vi "Write Key Value Boolean.vi"(7 "Section Name":string, 8 "error in (no error)":errorcluster, 9 "Value":bool, 10 "Key Name":string, 11 "Ini-File in":refnum<class "Ini-File.lvclass">) -> (0 "error out":errorcluster, 2 "found":bool, 3 "Ini-File out":refnum<class "Ini-File.lvclass">)   [LabVIEW 2016, in "Configuration.lvlib" / "Ini-File.lvclass"]
doc: "Write boolean value."
uses:
  Ini-File.lvclass
  Ini-File.lvclass/Ini-File.ctl
  <vilib>/Utility/config.llb/Write Key (Boolean).vi
  <vilib>/Utility/config.llb/NI_LVConfig.lvlib
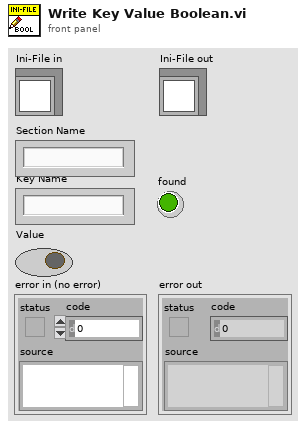
[diagram p1: front panel]
types:
  T1 = typedef "NI_LVConfig.lvlib/Config Data RefNum.ctl" = refnum<k1>
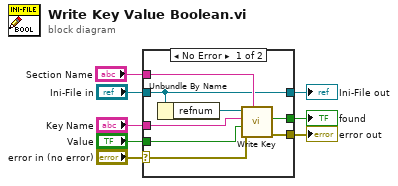
[diagram p0: block diagram]
diagram:
  n1 = case shown="No Error" "error in (no error)" {
    selector: "error in (no error)" -> [w9 w17]
    tunnel: "Ini-File in" -> [w10 w18]
    tunnel: "Section Name" -> [w15 _]
    tunnel: "Key Name" -> [w14 _]
    tunnel: "Value" -> [w13 _]
    tunnel: [w12 w17] -> w4
    tunnel: [w11 _] -> w3
    tunnel: [w10 w18] -> w2
    frame No Error {
      n2 = Unbundle By Name(w10) -> ("refnum"=w16:T1)
      n3 = call-poly <vilib>:"Write Key.vi"("section"=w15, "error in (no error)"=w9, "value"=w13, "key"=w14, "refnum"=w16) -> ("error out"=w12:errorcluster, "found?"=w11:bool)  [unwired: 4 in, 1 out]
    }
    frame Error {
    }
  }
  "error out" <- w4
  "Ini-File out" <- w2
  "found" <- w3
